vi "q_estimate.vi"(0 "new_offset":bool, 5 "feedback_time (ms)":fxp<+,16,1>, 7 "Q1_init":fxp<+/-,32,16>, 9 "Q2_init":fxp<+/-,32,16>, 11 "Q3_init in":fxp<+/-,32,16>, 12 "Q4_init in":fxp<+/-,32,16>) -> (4 "Q1 temp":fxp<+/-,32,16>, 6 "Q2 temp":fxp<+/-,32,16>, 10 "Q3_temp":fxp<+/-,32,16>, 13 "q1_valid":bool, 14 "Q2_valid":bool, 15 "Q4_temp":fxp<+/-,32,16>)   [LabVIEW 2020]
uses:
  <vilib>/rvi/FXPMathLib/FxpMul/XNode/nifxpmath_Multiplier.xnode
  <vilib>/rvi/FXPMathLib/FxpAdd/XNode/nifxpmath_Add.xnode
  <vilib>/rvi/FXPMathLib/sim/FxpSim.dll
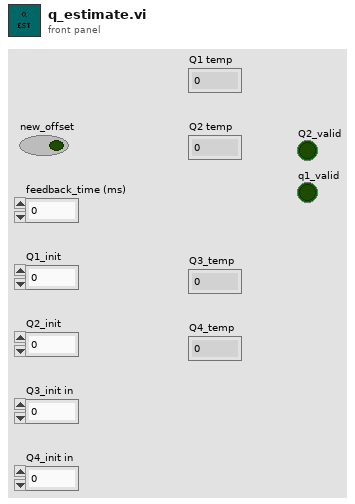
[diagram p1: front panel]
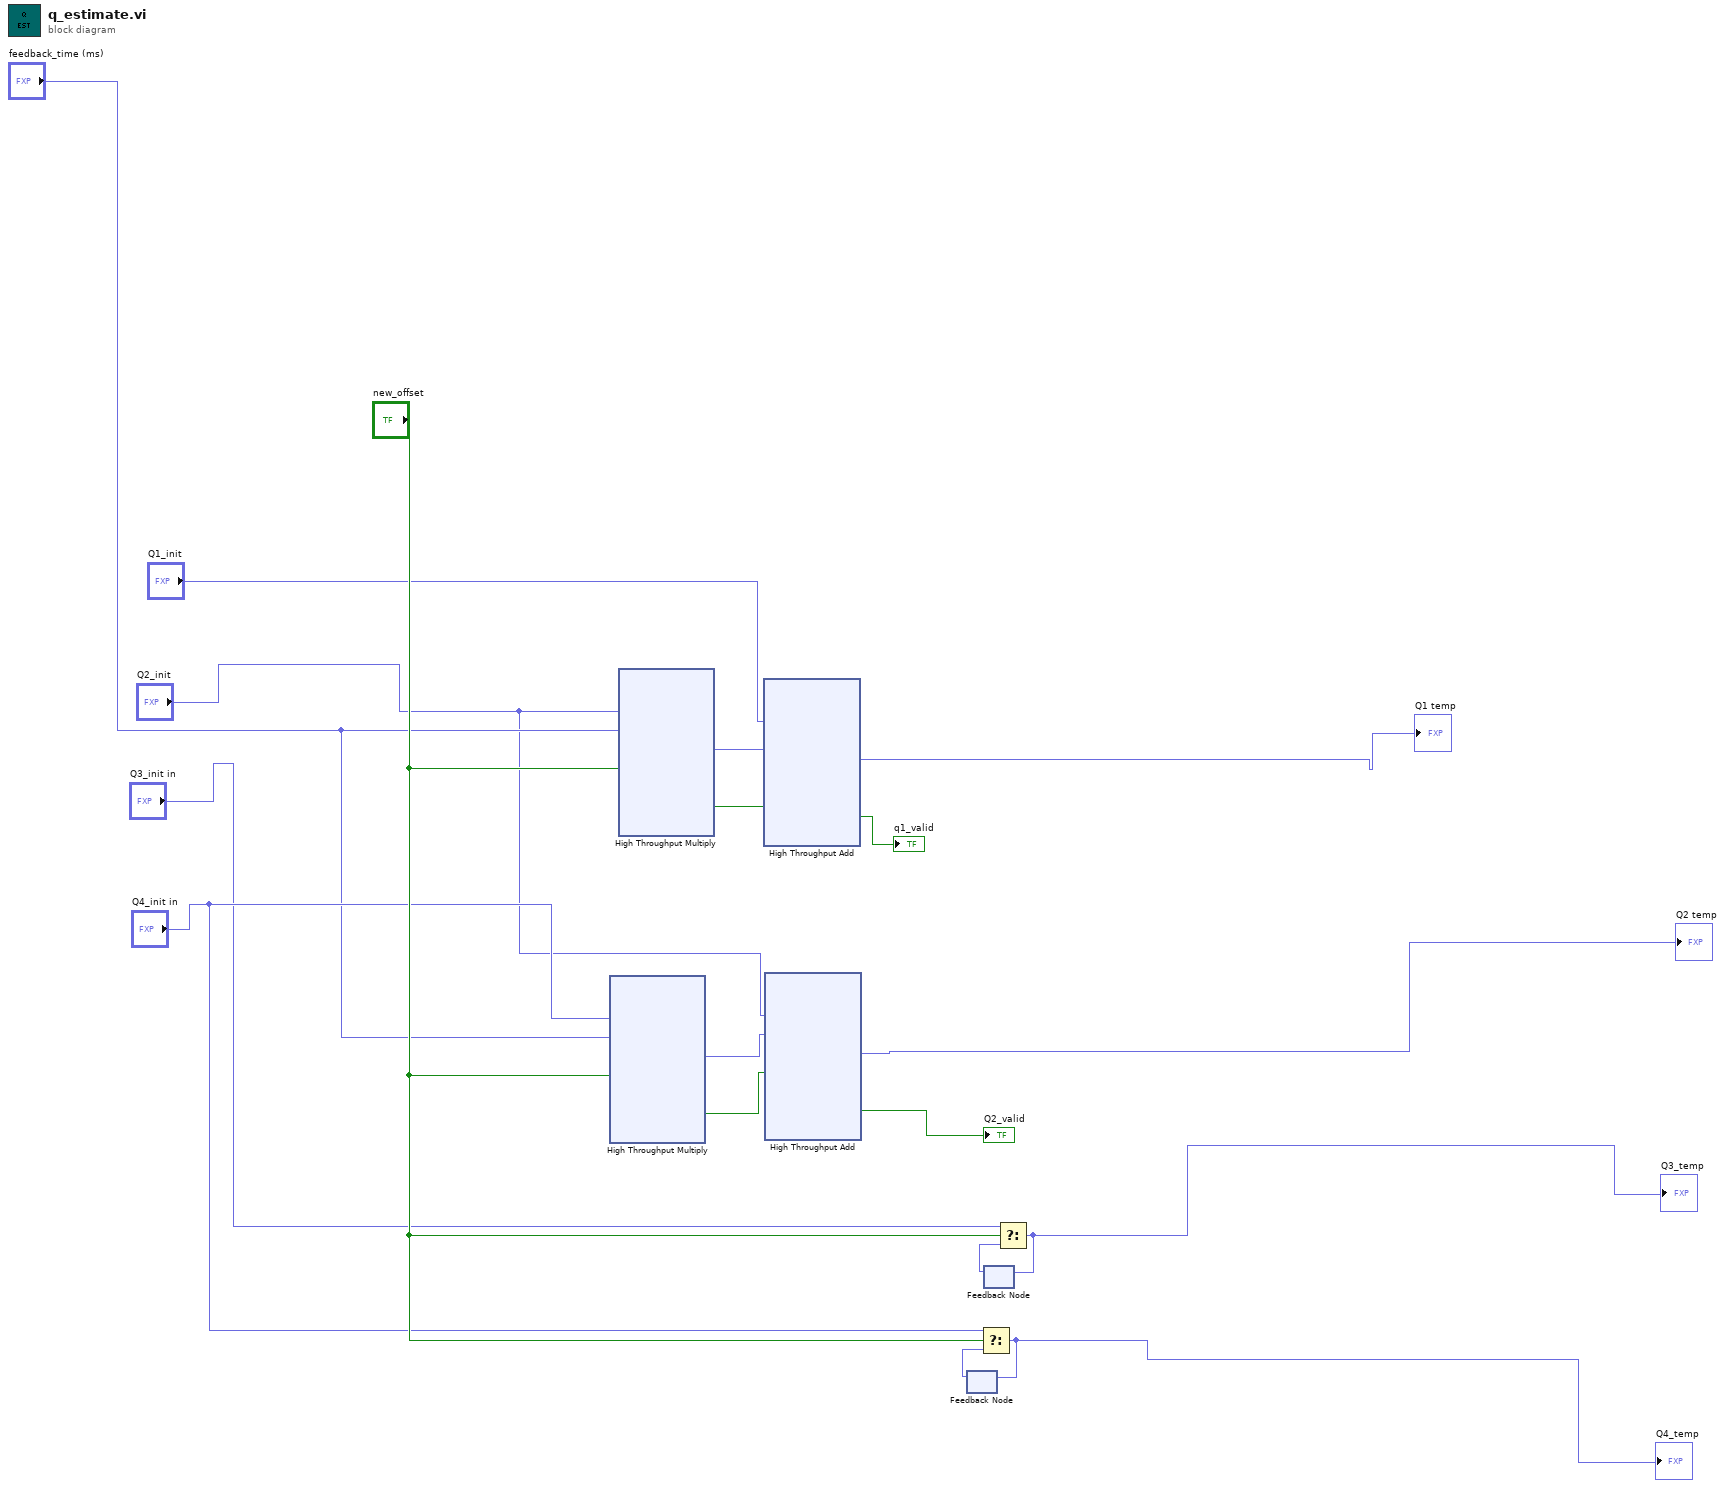
[diagram p0: block diagram]
diagram:
  n1 = xnode "High Throughput Multiply"("x"="Q4_init in", "y"="feedback_time (ms)", "input valid"="new_offset") -> ("x*y"=w11:fxp<+/-,32,16>, "output valid"=w12:bool)  [unwired: 1 in, 1 out]
  n2 = xnode "High Throughput Multiply"("x"="Q2_init", "y"="feedback_time (ms)", "input valid"="new_offset") -> ("x*y"=w9:fxp<+/-,32,16>, "output valid"=w10:bool)  [unwired: 1 in, 1 out]
  n3 = xnode "High Throughput Add"("x"="Q1_init", "y"=w9, "input valid"=w10) -> ("x+y"=→"Q1 temp":fxp<+/-,32,16>, "output valid"=→"q1_valid":bool)  [unwired: 1 in, 1 out]
  n4 = xnode "High Throughput Add"("x"="Q2_init", "y"=w11, "input valid"=w12) -> ("x+y"=→"Q2 temp":fxp<+/-,32,16>, "output valid"=→"Q2_valid":bool)  [unwired: 1 in, 1 out]
  n5 = feedback #1() -> (w16:fxp<+/-,32,16>)  [unwired: 1 in]
  n6 = Select(t="Q4_init in", s="new_offset", f=w16) -> (s? t:f=w6:fxp<+/-,32,16>)
  "Q4_temp" <- w6
  n7 = feedback-in #1(w6) -> ()
  n8 = feedback #2() -> (w15:fxp<+/-,32,16>)  [unwired: 1 in]
  n9 = Select(t="Q3_init in", s="new_offset", f=w15) -> (s? t:f=w7:fxp<+/-,32,16>)
  "Q3_temp" <- w7
  n10 = feedback-in #2(w7) -> ()
